vi "Get Section Content.vi"(10 "Section Name":string, 11 "INI in":refnum<class "LabVIEW-Config.lvclass">) -> (2 "Array":string[](array[string]), 3 "INI out":refnum<class "LabVIEW-Config.lvclass">)   [LabVIEW 2017, in "LabVIEW-Config.lvlib" / "LabVIEW-Config.lvclass"]
uses:
  LabVIEW-Config.lvclass
  LabVIEW-Config.lvclass/LabVIEW-Config.ctl
  14bbe030-ca6c-4c37-9b41-f1866c1e1f7f.vi
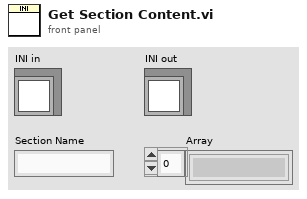
[diagram p1: front panel]
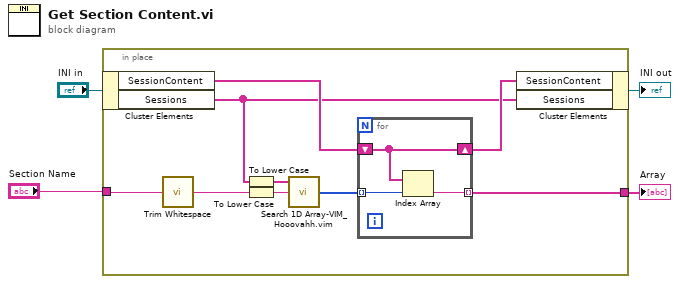
[diagram p0: block diagram]
diagram:
  n1 = in-place {
    in-place-border: "Section Name" -> [w7]
    in-place-border: [w5] -> w4
    n2 = in-place-cluster #1("INI in") -> ("SessionContent"=w10:string[], "Sessions"=w8:string[])
    n3 = call <vilib>:"Trim Whitespace.vi"("string"=w7) -> ("trimmed string"=w6:string)  [unwired: 1 in]
    n4 = To Lower Case(string=w8) -> (all lower case string=w12:string[])
    n5 = To Lower Case(string=w6) -> (all lower case string=w13:string)
    n6 = call "Search 1D Array-VIM_Hooovahh.vim"("Array"=w12, "Element Data"=w13) -> ("Indices of Elements"=w11:i32[])  [unwired: 7 in]
    n7 = for {
      shift-right: [w16] -> w9
      shift-left: w10 -> [w16]
      tunnel: w11 -> [w15] mode=indexing
      tunnel: [w14] -> w5 mode=indexing
      n8 = Index Array(array=w16, index=w15) -> (element=w14:string)
    }
    n9 = in-place-cluster #1("SessionContent"=w9, "Sessions"=w8) -> (→"INI out":refnum<class "LabVIEW-Config.lvclass">)
  }
  "Array" <- w4
